vi "tearDown.vi"(8 "error in (no error)":errorcluster, 11 "TestCaseErrors":refnum<class "TestCaseErrors.lvclass">) -> (0 "error out":errorcluster, 3 "TestCaseErrors out":refnum<class "TestCaseErrors.lvclass">)   [LabVIEW 2013, in "TestCaseErrors.lvclass"]
uses:
  TestCaseErrors.lvclass
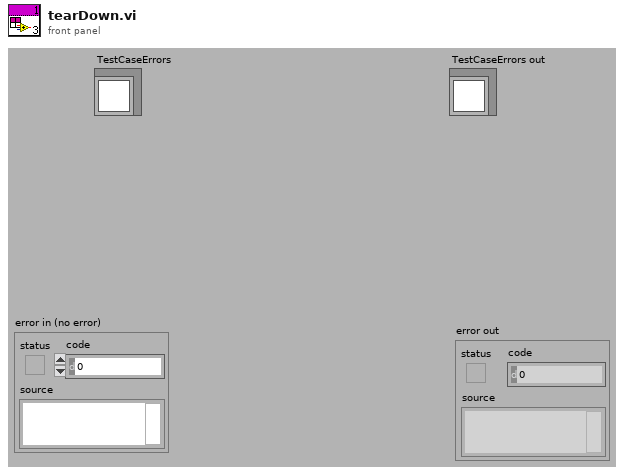
[diagram p1: front panel]
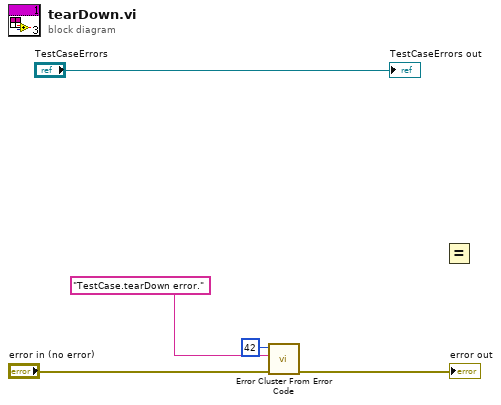
[diagram p0: block diagram]
diagram:
  n1 = call <vilib>:"Error Cluster From Error Code.vi"("error in (no error)"="error in (no error)", "error message (\"\")"="TestCase.tearDown error." ("error message (\"\")"), "error code (0)"=42) -> ("error out"=→"error out":errorcluster)  [unwired: 6 in]
  n2 = Equal?() -> ()  [unwired: 2 in, 1 out]
  "TestCaseErrors out" <- "TestCaseErrors"
